vi "Load Image from File.vi"(8 "error in (no error)":errorcluster, 9 "Load Report":bool, 10 "Image":path, 11 "HIJ Vision File Viewer in":refnum<class "HIJ Vision File Display.lvclass">) -> (0 "error out":errorcluster, 3 "HIJ Vision File Viewer out":refnum<class "HIJ Vision File Display.lvclass">)   [LabVIEW 2014, in "HIJ Vision File Display.lvlib" / "HIJ Vision File Display.lvclass"]
uses:
  HIJ Vision File Display.lvclass
  HIJ Vision File Display.lvclass/HIJ Vision File Display.ctl
  HIJ Vision Display/HIJ Vision Display/HIJ Vision Display.lvclass/HIJ Vision Display.ctl
  HIJ Vision Display/HIJ Vision Display/Read Display Image.vi
  HIJ Vision Display/HIJ Vision Display/Write WorkDir.vi
  HIJ Vision Display/HIJ Vision Display/Write Image Source Name.vi
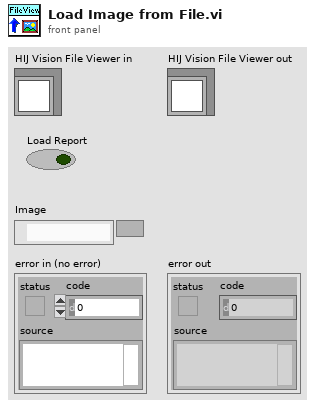
[diagram p1: front panel]
types:
  T1 = typedef "IMAQ Image.ctl" = refnum<image>
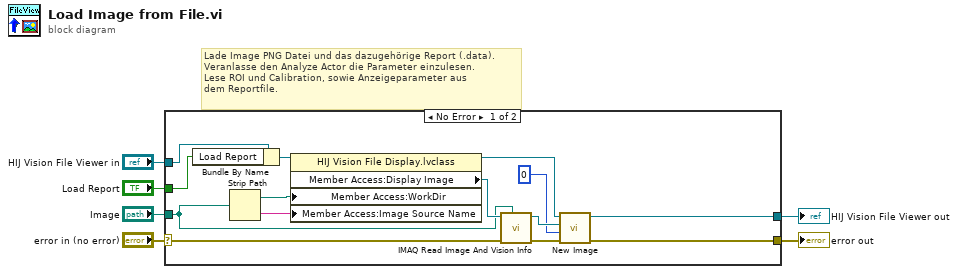
[diagram p0: block diagram]
diagram:
  # "Lade Image PNG Datei und das dazugehörige Report (.data).\nVeranlasse den Analyze Actor die Parameter einzulesen.\nLese ROI und Calibration, sowie Anzeigeparameter aus\ndem Reportfile."
  n1 = case shown="No Error" "error in (no error)" {
    selector: "error in (no error)" -> [w15 w22]
    tunnel: [w14 w22] -> w5
    tunnel: [w12 w21] -> w3
    tunnel: "HIJ Vision File Viewer in" -> [w16 w21]
    tunnel: "Image" -> [w9 _]
    tunnel: "Load Report" -> [w7 _]
    frame No Error {
      n2 = Bundle By Name(cluster=w16, "Load Report"=w7) -> (w8:refnum<class "HIJ Vision File Display.lvclass">)
      n3 = Strip Path(path=w9) -> (stripped path=w11:path, name=w10:string)
      n4 = property class="HIJ Vision File Display.lvclass"(reference=w8, "Member Access:WorkDir"=w11, "Member Access:Image Source Name"=w10) -> (reference out=w13:refnum<class "HIJ Vision File Display.lvclass">, "Member Access:Display Image"=w20:T1)  [unwired: 1 in, 1 out]
      n5 = call "IMAQ Read Image And Vision Info"("File Path"=w9, "error in (no error)"=w15, "Image"=w20) -> ("error out"=w18:errorcluster, "Image Out"=w19:T1)  [unwired: 6 in, 1 out]
      n6 = call-dynamic "New Image.vi"("error in (no error)"=w18, "Buffer Number"=0, "Image"=w19, "IMAQ Display in"=w13) -> ("error out"=w14:errorcluster, "IMAQ Display out"=w12:refnum<class "HIJ Vision File Display.lvclass">)  [unwired: 6 in]
    }
    frame Error {
    }
  }
  "error out" <- w5
  "HIJ Vision File Viewer out" <- w3
